vi "Identities.vi"(8 "error in (no error)":errorcluster, 11 "DataHandlerAPI in":refnum<class "DataHandlerAPI.lvclass">) -> (0 "error out":errorcluster, 2 "Identities":refnum<class "Identity.lvclass">[](array[class]), 3 "DataHandlerAPI out":refnum<class "DataHandlerAPI.lvclass">)   [LabVIEW 2020, in "VolatusData.lvlib" / "DataHandlerAPI.lvclass"]
uses:
  DataHandlerAPI.lvclass
  DataHandlerIdentity/DataHandlerIdentity.lvclass
  C:/dev/lv20CE/relink/lv-volatus/Volatus/DataHandlerIdentity/DataHandlerIdentity.lvclass
  C:/dev/lv20CE/relink/lv-volatus/Volatus/Identity/Identity.lvclass
  Volatus/Identity/Identity.lvclass
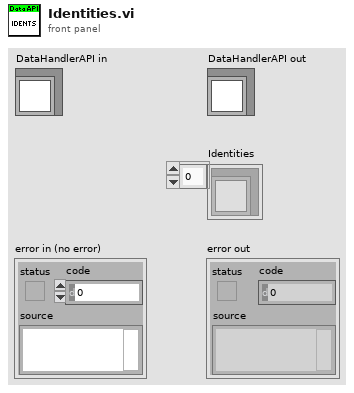
[diagram p1: front panel]
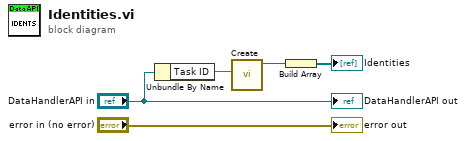
[diagram p0: block diagram]
diagram:
  n1 = Unbundle By Name("DataHandlerAPI in") -> ("Task ID"=w1:string)
  n2 = call "Create.vi"("Task ID"=w1) -> ("DataHandlerIdentity out"=w3:refnum<class "DataHandlerIdentity.lvclass">)  [unwired: 10 in]
  n3 = Build Array(w3) -> (→"Identities":refnum<class "DataHandlerIdentity.lvclass">[])
  "error out" <- "error in (no error)"
  "DataHandlerAPI out" <- "DataHandlerAPI in"
